vi "Route and Generate Sync Pulse.vi"(0 "fpga interfaces in":refnum<k20>[](array[refnum]), 5 "sync pulse sender index":i32, 7 "sync pulse source terminal":string="/SyncPulseSource", 9 "sync pulse destination terminal":string="/SyncPulseDestination", 11 "error in (no error)":errorcluster) -> (4 "fpga interfaces out":refnum<k20>[](array[refnum]), 15 "error out":errorcluster)   [LabVIEW 2023, in "GettingStarted_Common_148X_Host.lvlib"]
uses:
  GettingStarted_Common_148X_Host.lvlib
  Types/148x_Common_FPGA_Reference.ctl
  <vilib>/Utility/error.llb/Error Cluster From Error Code.vi
  <vilib>/rvi/errors/niLvFpgaAdjustHostInterfaceError.vi
  <vilib>/rvi/interface/nirviReadWriteControl/nirviReadWriteControl.xnode
  <instrlib>/FlexRIO/API/Host/v1/NI FlexRIO API v1.lvlib
  <vilib>/rvi/interface/Simulation/niFpgaSimulationCallBeginRW.vi
  NiFpgaLv.dll
  <instrlib>/FlexRIO/Automotive Vision Utility/v1/Host/Automotive Vision Utility.lvlib
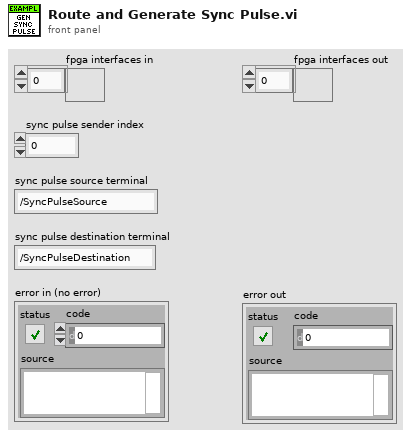
[diagram p1: front panel]
types:
  T1 = typedef "GettingStarted_Common_148X_Host.lvlib/148x_Common_FPGA_Reference.ctl" = refnum<k20>
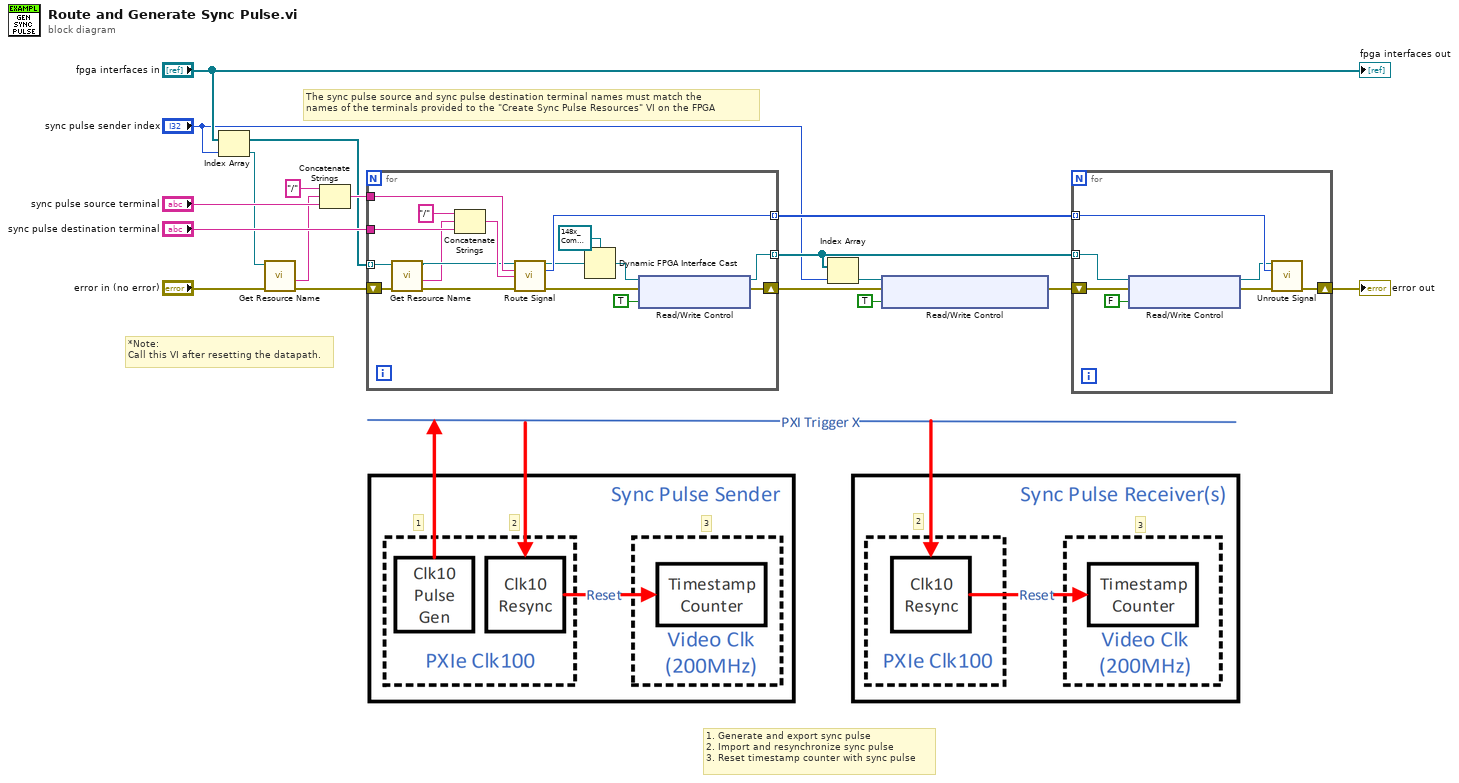
[diagram p0: block diagram]
diagram:
  # "*Note: \nCall this VI after resetting the datapath."
  # "1. Generate and export sync pulse\n2. Import and resynchronize sync pulse\n3. Reset timestamp counter with sync pulse"
  # "3"
  # "2"
  # "3"
  # "2"
  # "1"
  # "The sync pulse source and sync pulse destination terminal names must match the \nnames of the terminals provided to the \"Create Sync Pulse Resources\" VI on the FPGA"
  n1 = Index Array(array="fpga interfaces in", index="sync pulse sender index") -> (element=w1:refnum<k20>)
  n2 = call <instrlib>:"Get Resource Name.vi"("error in"="error in (no error)", "fpga interface in"=w1) -> ("error out"=w3:errorcluster, "alias"=w2:string)  [unwired: 6 in, 2 out]
  n3 = Concatenate Strings("/" ("string"), w2, "sync pulse source terminal") -> (w11:string)
  n4 = for {
    tunnel: w11 -> [w34]
    tunnel: [w31] -> w12 mode=indexing
    tunnel: [w28] -> w16 mode=indexing
    shift-right: [w29] -> w9
    shift-left: w3 -> [w22]
    tunnel: "fpga interfaces in" -> [w19] mode=indexing
    tunnel: "sync pulse destination terminal" -> [w26]
    n5 = call <instrlib>:"Get Resource Name.vi"("error in"=w22, "fpga interface in"=w19) -> ("error out"=w21:errorcluster, "alias"=w18:string, "fpga interface out"=w20:refnum<k20>)  [unwired: 6 in, 1 out]
    n6 = Concatenate Strings("/" ("string"), w18, w26) -> (w32:string)
    n7 = call <instrlib>:"Route Signal.vi"("fpga interface in"=w20, "source"=w34, "destination"=w32, "error in"=w21) -> ("fpga interface out"=w24:refnum<k20>, "route ticket"=w31:u32, "error out"=w30:errorcluster)  [unwired: 9 in]
    n8 = Dynamic FPGA Interface Cast(Session In=T1 refnum ("FPGA VI Reference Out"), Type=w24) -> (Session Out=w23:T1)
    n9 = xnode "Read/Write Control"("FPGA VI Reference In"=w23, "error in"=w30, "enable sync pulse"=TRUE ("enable sync pulse reset")) -> ("FPGA VI Reference Out"=w28:T1, "error out"=w29:errorcluster)
  }
  n10 = Index Array(array=w16, index="sync pulse sender index") -> (element=w15:T1)
  n11 = xnode "Read/Write Control"("FPGA VI Reference In"=w15, "error in"=w9, "generate sync pulse (strobe)"=TRUE ("generate clk10  pulse (strobe)")) -> ("error out"=w13:errorcluster)  [unwired: 1 out]
  n12 = for {
    shift-right: [w41] -> w17
    shift-left: w13 -> [w38]
    tunnel: w12 -> [w40] mode=indexing
    tunnel: w16 -> [w35] mode=indexing
    n13 = xnode "Read/Write Control"("FPGA VI Reference In"=w35, "error in"=w38, "enable sync pulse"=FALSE ("enable sync pulse reset")) -> ("FPGA VI Reference Out"=w36:T1, "error out"=w37:errorcluster)
    n14 = call <instrlib>:"Unroute Signal.vi"("fpga interface in"=w36, "route ticket"=w40, "error in"=w37) -> ("error out"=w41:errorcluster)  [unwired: 11 in, 1 out]
  }
  "error out" <- w17
  "fpga interfaces out" <- "fpga interfaces in"
